vi "Translate_MULTICOLUMNLISTBOX.vi"(8 "error IN":errorcluster, 10 "Cle":string, 11 "MCListbox Refnum":refnum<vi>) -> (0 "error out":errorcluster)   [LabVIEW 2011]
uses:
  Dictionnary/EnumCommandDictionnaire.ctl
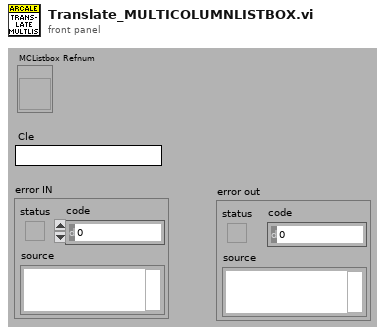
[diagram p1: front panel]
types:
  T1 = typedef "EnumCommandDictionnaire.ctl" = enum16{"Load", "Translate", "Save", "GetDico", "Set : A traduire = Vrai", "Set : A Traduire = Faux", "SetDico"}
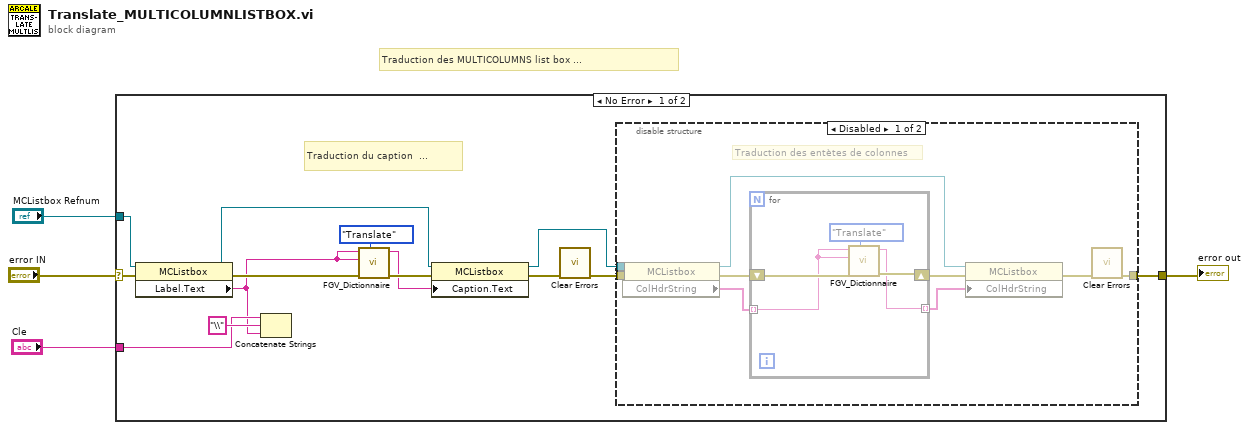
[diagram p0: block diagram]
diagram:
  # "Traduction des MULTICOLUMNS list box ..."
  n1 = case shown="No Error" "error IN" {
    selector: "error IN" -> [w18 w34]
    tunnel: "MCListbox Refnum" -> [w17 _]
    tunnel: "Cle" -> [w13 _]
    tunnel: [w5 w34] -> w1
    frame No Error {
      # "Traduction du caption  ..."
      n2 = property class="MCListbox"(reference=w17, error in=w18) -> (reference out=w14:refnum<vi>, error out=w11:errorcluster, "Label.Text"=w8:string)
      n3 = Concatenate Strings(w13, "\\" ("string"), w8) -> ()  [unwired: 1 out]
      n4 = call "FGV_Dictionnaire.vi"("Command"=EnumCommandDictionnaire."Translate", "error in (no error)"=w11, "Chaîne"=w8, "Clé"=w8) -> ("error out"=w10:errorcluster, "Traduction"=w9:string)  [unwired: 5 in, 1 out]
      n5 = property class="MCListbox"(reference=w14, error in=w10, "Caption.Text"=w9) -> (reference out=w6:refnum<vi>, error out=w15:errorcluster)
      n6 = call <vilib>:"Clear Errors.vi"("error in (no error)"=w15) -> ("error out"=w7:errorcluster)  [unwired: 6 in]
      n7 = disable-structure shown="Disabled" {
        disable-tunnel: w7 -> [w27 w33]
        disable-tunnel: w6 -> [w26 _]
        disable-tunnel: [w19 w33] -> w5
        frame Disabled {
          # "Traduction des entètes de colonnes"
          n8 = property class="MCListbox"(reference=w26, error in=w27) -> (reference out=w21:refnum<vi>, error out=w25:errorcluster, "ColHdrString"=w24:string[])
          n9 = for {
            shift-right: [w30] -> w23
            shift-left: w25 -> [w31]
            tunnel: w24 -> [w29] mode=indexing
            tunnel: [w28] -> w22 mode=indexing
            n10 = call "FGV_Dictionnaire.vi"("Command"=EnumCommandDictionnaire."Translate", "error in (no error)"=w31, "Chaîne"=w29, "Clé"=w29) -> ("error out"=w30:errorcluster, "Traduction"=w28:string)  [unwired: 5 in, 1 out]
          }
          n11 = property class="MCListbox"(reference=w21, error in=w23, "ColHdrString"=w22) -> (error out=w20:errorcluster)  [unwired: 1 out]
          n12 = call <vilib>:"Clear Errors.vi"("error in (no error)"=w20) -> ("error out"=w19:errorcluster)  [unwired: 6 in]
        }
        frame Enabled {
        }
      }
    }
    frame Error {
    }
  }
  "error out" <- w1
